vi "PathPlanner_CommandUtil_Equals.vi"(9 "Other EventMarker":T1, 11 "Command":T1) -> (3 "Equal":bool)   [LabVIEW 2019, in "PathPlanner24.lvlib"]
doc: "Determines if two Command definitions are equal\n\nInputs:\n -- Command - cluster - command definition\n -- Other Command - cluster - command definition\n\nOutputs:\n -- Equal - boolean - TRUE if both definitions are the same."
uses:
  PathPlanner24.lvlib
  TypeDef/PathPlannerCommandUtil.ctl
  ENum/PathPlanner_CommandUtilType_ENUM.ctl
  <vilib>/Rock Robotics/WPI/ThirdParty/JAS_Junk/TrajLib/Trajectory_Library.lvlib
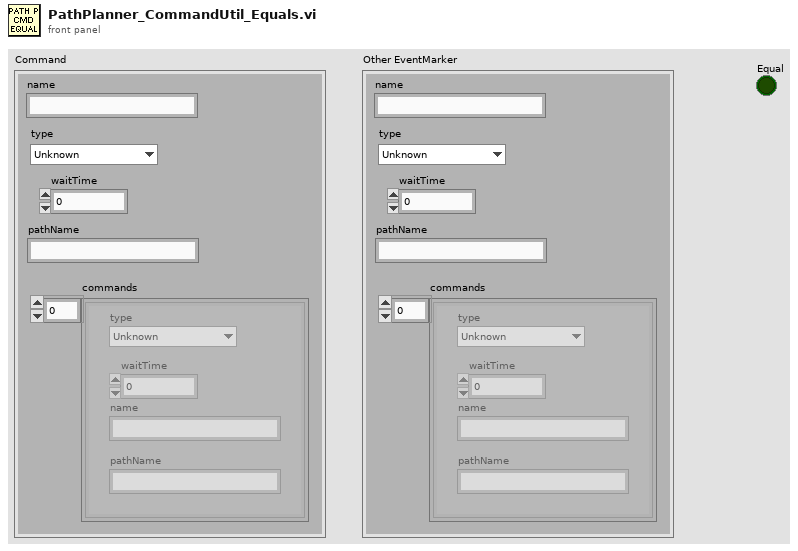
[diagram p1: front panel]
types:
  T1 = typedef "PathPlanner24.lvlib/PathPlannerCommandUtil.ctl" = cluster{"waitTime":dbl, "name":string, "pathName":string, "commands":cluster{"type":T2, "waitTime":dbl, "name":string, "pathName":string}[], "type":T2}
  T2 = typedef "PathPlanner24.lvlib/PathPlanner_CommandUtilType_ENUM.ctl" = enum16{"Unknown", "Wait", "Named", "Path", "Sequential", "Parallel", "Race", "Deadline"}
  T3 = cluster{"type":T2, "waitTime":dbl, "name":string, "pathName":string}[]
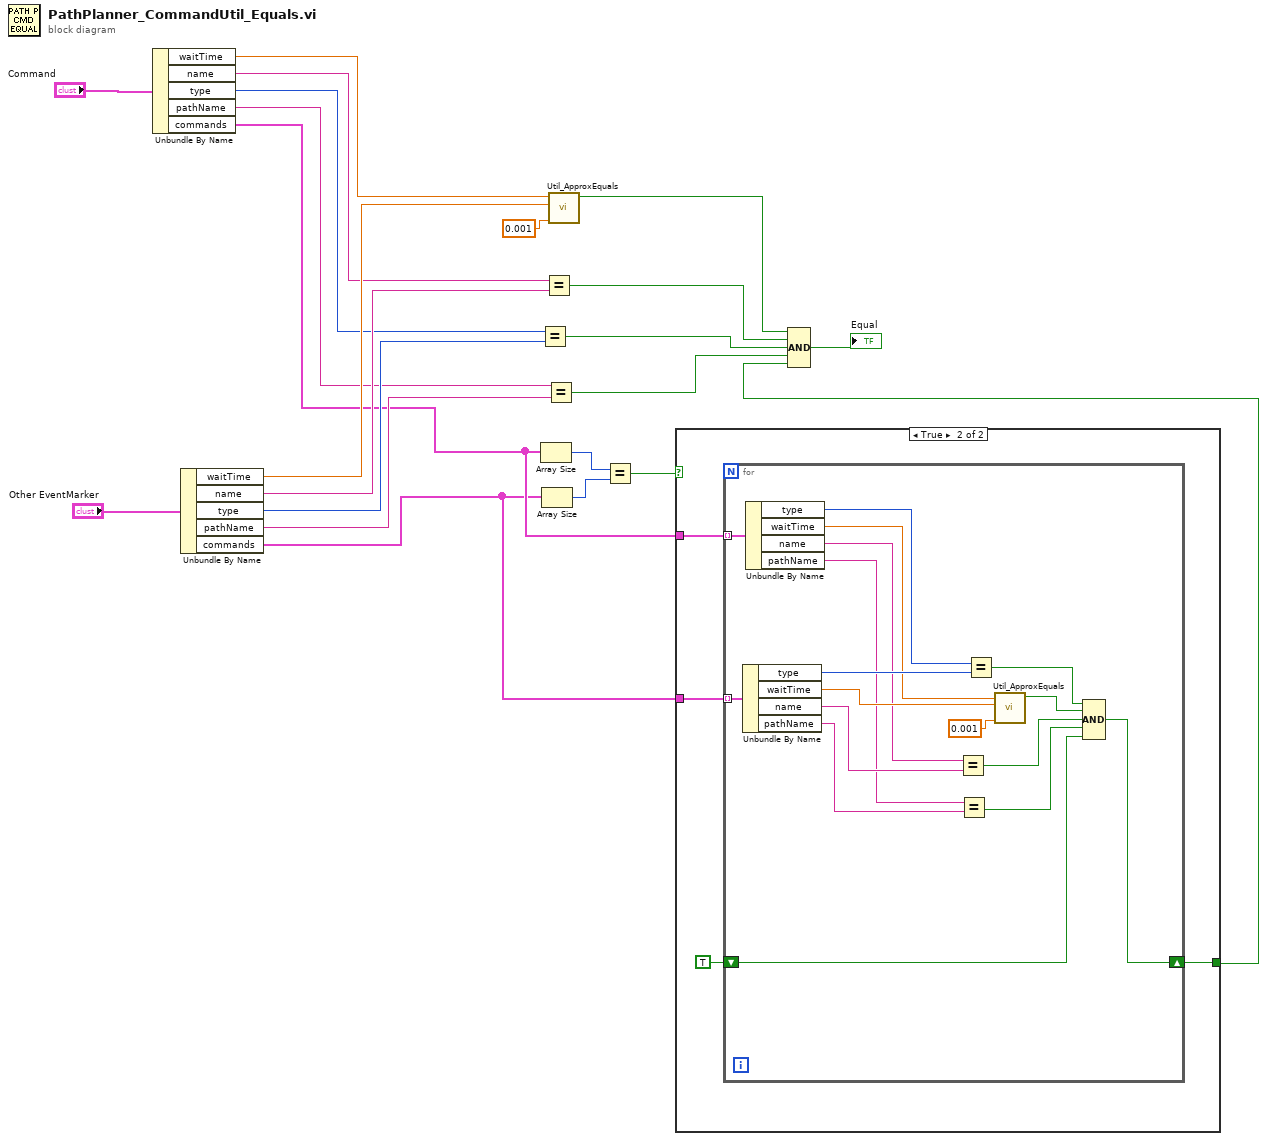
[diagram p0: block diagram]
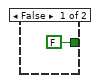
[diagram p2: hidden frame]
diagram:
  n1 = Unbundle By Name("Command") -> ("waitTime"=w18:dbl, "name"=w15:string, "type"=w13:T2, "pathName"=w11:string, "commands"=w3:T3)
  n2 = Unbundle By Name("Other EventMarker") -> ("waitTime"=w17:dbl, "name"=w14:string, "type"=w12:T2, "pathName"=w10:string, "commands"=w2:T3)
  n3 = Equal?(x=w13, y=w12) -> (x = y?=w8:bool)
  n4 = Array Size(array=w3) -> (size(s)=w6:i32)
  n5 = Array Size(array=w2) -> (size(s)=w5:i32)
  n6 = Equal?(x=w15, y=w14) -> (x = y?=w9:bool)
  n7 = Equal?(x=w11, y=w10) -> (x = y?=w7:bool)
  n8 = call <vilib>:"Util_ApproxEquals.vi"("Tolerance"=0.001 ("y"), "Value 2"=w17, "Value 1"=w18) -> ("ApproxEquals"=w16:bool)  [unwired: 8 in]
  n9 = Equal?(x=w6, y=w5) -> (x = y?=w4:bool)
  n10 = case shown="True" w4 {
    tunnel: w3 -> [_ w27]
    tunnel: w2 -> [_ w26]
    tunnel: [FALSE w24] -> w1
    frame False {
    }
    frame True {
      n11 = for {
        tunnel: w27 -> [w44] mode=indexing
        tunnel: w26 -> [w43] mode=indexing
        shift-right: [w28] -> w24
        shift-left: TRUE -> [w29]
        n12 = Unbundle By Name(w43) -> ("type"=w40:T2, "waitTime"=w38:dbl, "name"=w36:string, "pathName"=w34:string)
        n13 = Unbundle By Name(w44) -> ("type"=w41:T2, "waitTime"=w39:dbl, "name"=w37:string, "pathName"=w35:string)
        n14 = Equal?(x=w37, y=w36) -> (x = y?=w31:bool)
        n15 = Equal?(x=w35, y=w34) -> (x = y?=w30:bool)
        n16 = Equal?(x=w41, y=w40) -> (x = y?=w33:bool)
        n17 = call <vilib>:"Util_ApproxEquals.vi"("Tolerance"=0.001 ("y"), "Value 2"=w38, "Value 1"=w39) -> ("ApproxEquals"=w32:bool)  [unwired: 8 in]
        n18 = Compound Arithmetic op=AND(w33, w32, w31, w30, w29) -> (w28:bool)
      }
    }
  }
  n19 = Compound Arithmetic op=AND(w16, w9, w8, w7, w1) -> (→"Equal":bool)
